vi "WaitBallOrientSkill.vi"(6 "Role ofRobotThat\nmake the pass":T1=enum."PassKicker", 8 "error in (no error)":errorcluster, 9 "Robot":refnum<class "Robot.lvclass">, 10 "Game":refnum<class "Game.lvclass">, 11 "WaitBallOrientSkill in":refnum<class "WaitBallOrientSkill.lvclass">) -> (0 "error out":errorcluster, 2 "robot out":refnum<class "Robot.lvclass">, 3 "WaitBallOrientSkill out":refnum<class "WaitBallOrientSkill.lvclass">)   [LabVIEW 2024, in "WaitBallOrientSkill.lvclass"]
uses:
  WaitBallOrientSkill.lvclass
  Robot_class/Robot.lvclass
  C:/Users/moise/Documents/GitHub/SSL_AI/Object_class/Object.lvclass
  Game_class/Game.lvclass
  Robot_class/roles.ctl
  Object_class/Object.lvclass/Object.ctl
  Game_class/Game.lvclass/Game.ctl
  Team_class/Team.lvclass/Team.ctl
  Robot_class/Robot.lvclass/Robot.ctl
  Game_class/Read BallRef.vi
  Game_class/Read Utilities.lvclass.vi
  Game_class/Read FieldRef.vi
  Game_class/Read OffensiveTeam.vi
  Team_class/Read RobotRef.vi
  Object_class/Read x.vi
  Object_class/Read y.vi
  Robot_class/Read orientation.vi
  Robot_class/Write dest_x.vi
  Robot_class/Write dest_y.vi
  Robot_class/Write dest_orientation.vi
  Ally_class/Ally.lvclass
  C:/Users/moise/Documents/GitHub/SSL_AI/Team_class/Team.lvclass
  Ball_class/Ball.lvclass
  Utilities_class/Utilities.lvclass
  Field_class/Field.lvclass
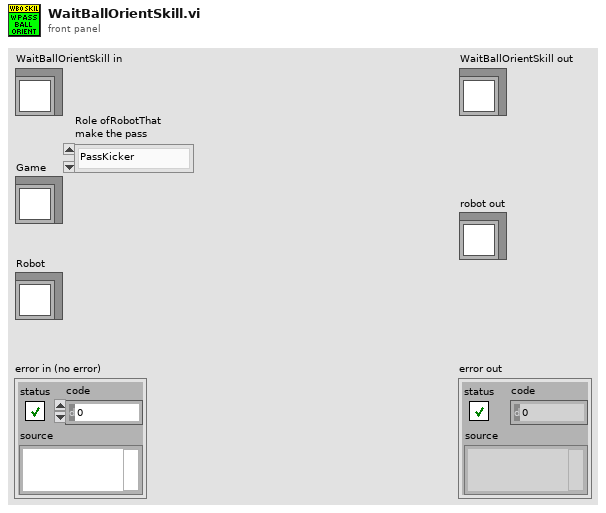
[diagram p1: front panel]
types:
  T1 = typedef "roles.ctl" = enum16{"SimpleBallPlacement", "BallPlacementAllyPasser", "BallPlacementAllyReceiver", "BallPlacementEnemy", "5Robots5th", "PassBestReceiver", "5Robots4th", "5Robots3rd", "5Robots2nd", "5Robots1st", "PassBestRobot", "WaitPass", "ABCThirdKicker", "ABCFirstKicker", "ABCSecondKicker", "Tabler", "TableFinalizer", "PrepareRollToPassRoller", "PrepareRollToPassReceiver", "SimplePassRoll", "SimplePassRollReceiver", "PenaltyDefense", "PreparePassReceiver 2", "PreparePassReceiver 1", "PassObserver", "Timeout", "Goto", "ZigZag", "None", "BallOutOfField", "DefenderArea", "Duelist", "AttackerStop", "FollowAttacker", "KeeperRole", "KickPenalty", "AttackerAimGoal", "AttackerBlock", "Marker", "Halt", "Shoot", "PassKicker", "PassReceiver", "TestRole", "PenaltyAttacker"}
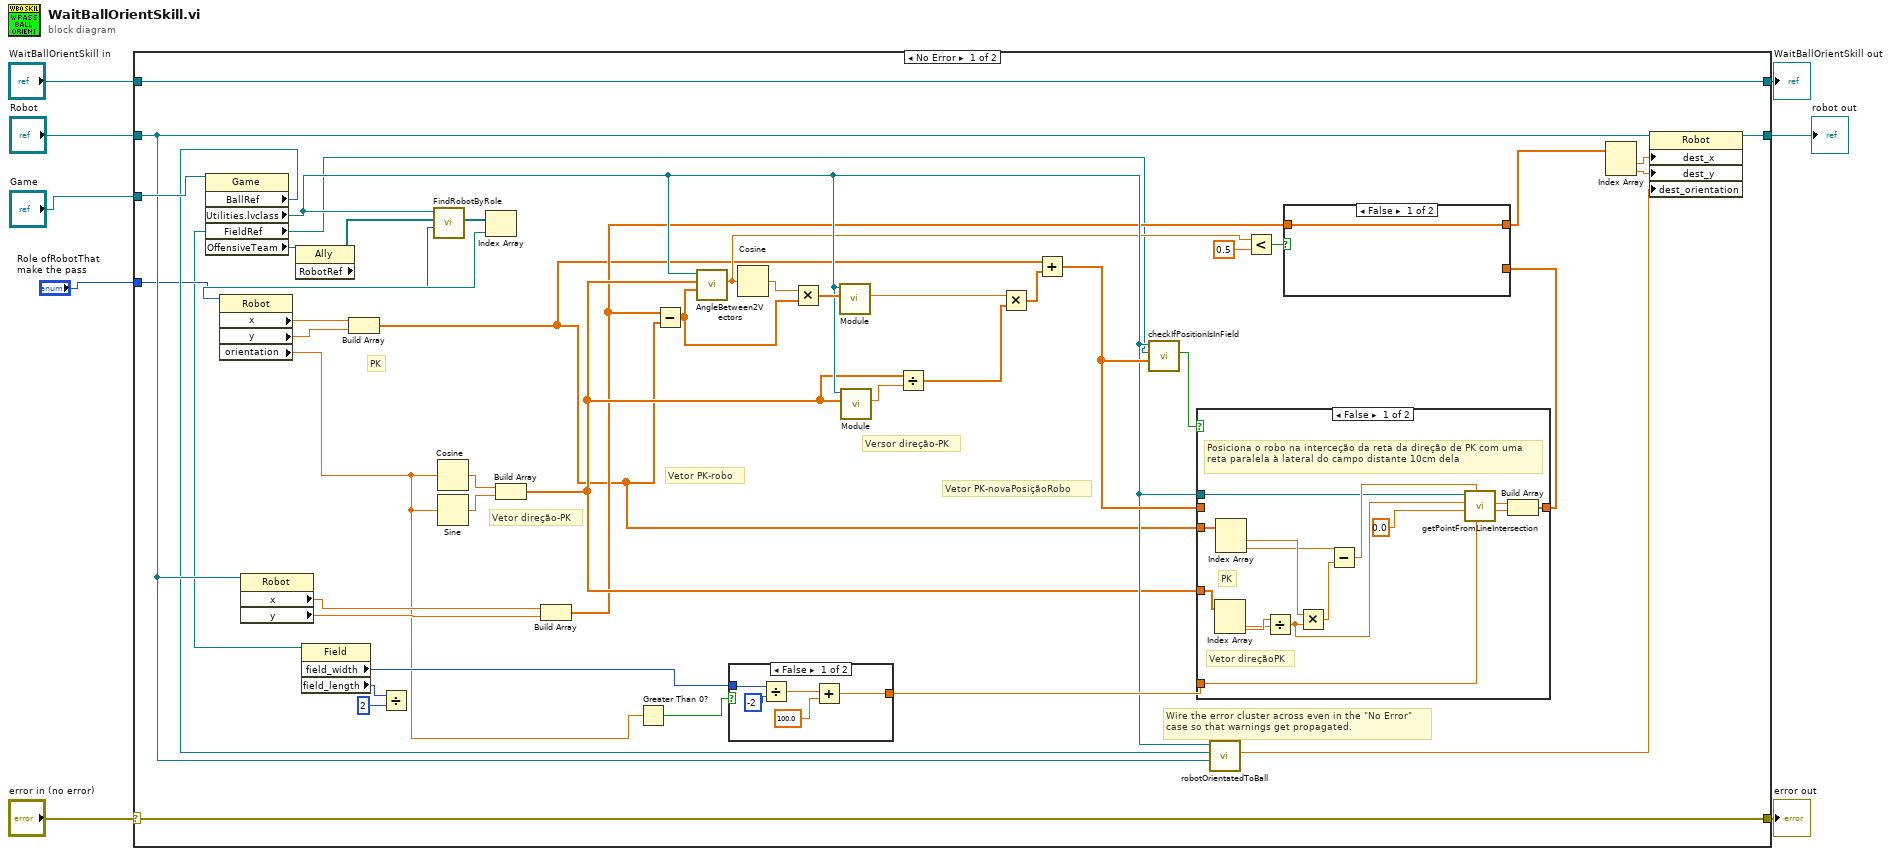
[diagram p0: block diagram]
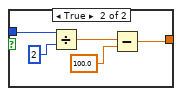
[diagram p4: hidden frame]
diagram:
  n1 = case shown="No Error" "error in (no error)" {
    selector: "error in (no error)" -> [w52 w83]
    tunnel: [w52 w83] -> w7
    tunnel: [w53 w82] -> w5
    tunnel: "WaitBallOrientSkill in" -> [w53 w82]
    tunnel: "Robot" -> [w29 _]
    tunnel: [w34 _] -> w3
    tunnel: "Game" -> [w30 _]
    tunnel: "Role ofRobotThat\nmake the pass" -> [w15 _]
    frame No Error {
      # "Versor direção-PK"
      # "PK"
      # "Vetor direção-PK"
      # "Vetor PK-novaPosiçãoRobo"
      # "Vetor PK-robo"
      # "Wire the error cluster across even in the \"No Error\"\ncase so that warnings get propagated."
      n2 = property class="Game"(reference=w30) -> ("BallRef"=w16:refnum<class "Ball.lvclass">, "Utilities.lvclass"=w25:refnum<class "Utilities.lvclass">, "FieldRef"=w13:refnum<class "Field.lvclass">, "OffensiveTeam"=w40:refnum<class "Ally.lvclass">)  [unwired: 1 in, 2 out]
      n3 = property class="Robot"(reference=w29) -> ("x"=w51:dbl, "y"=w50:dbl)  [unwired: 1 in, 2 out]
      n4 = property class="Ally"(reference=w40) -> ("RobotRef"=w39:refnum<class "Robot.lvclass">[])  [unwired: 1 in, 2 out]
      n5 = property class="Field"(reference=w13) -> ("field_width"=w44:i32, "field_length"=w12:i32)  [unwired: 1 in, 2 out]
      n6 = Divide(x=w12, y=2) -> ()  [unwired: 1 out]
      n7 = call "FindRobotByRole.vi"("role"=w15, "RobotRef"=w39, "Utilities in"=w25) -> ("Robots"=w37:refnum<class "Robot.lvclass">[])  [unwired: 5 in, 3 out]
      n8 = Index Array(array=w37) -> (element=w38:refnum<class "Robot.lvclass">)  [unwired: 1 in]
      n9 = property class="Robot"(reference=w38) -> ("x"=w36:dbl, "y"=w35:dbl, "orientation"=w31:dbl)  [unwired: 1 in, 2 out]
      n10 = Build Array(w36, w35) -> (w10:dbl[])
      n11 = Cosine(x=w31) -> (cos(x)=w33:dbl)
      n12 = Sine(x=w31) -> (sin(x)=w32:dbl)
      n13 = Build Array(w33, w32) -> (w23:dbl[])
      n14 = Build Array(w51, w50) -> (w19:dbl[])
      n15 = Greater Than 0?(x=w31) -> (x > 0?=w45:bool)
      n16 = Subtract(x=w19, y=w10) -> (x-y=w49:dbl[])
      n17 = call "AngleBetween2Vectors.vi"("Array 1"=w49, "Array 2"=w23, "Utilities in"=w25) -> ("angleInRadians(default)"=w20:dbl)  [unwired: 5 in, 3 out]
      n18 = case shown="False" w45 {
        tunnel: w44 -> [w75 w81]
        tunnel: [w74 w79] -> w43
        frame False {
          n19 = Divide(x=w75, y=-2) -> (x/y=w73:dbl)
          n20 = Add(x=w73, y=100.0) -> (x+y=w74:dbl)
        }
        frame True {
          n21 = Divide(x=w81, y=2) -> (x/y=w78:dbl)
          n22 = Subtract(x=w78, y=100.0) -> (x-y=w79:dbl)
        }
      }
      n23 = Cosine(x=w20) -> (cos(x)=w48:dbl)
      n24 = Multiply(x=w48, y=w49) -> (x*y=w28:dbl[])
      n25 = call "Module.vi"("2D vector"=w28, "Utilities in"=w25) -> ("Modulo"=w26:dbl)  [unwired: 7 in, 2 out]
      n26 = call "Module.vi"("2D vector"=w23, "Utilities in"=w25) -> ("Modulo"=w22:dbl)  [unwired: 7 in, 2 out]
      n27 = Divide(x=w23, y=w22) -> (x/y=w24:dbl[])
      n28 = Multiply(x=w26, y=w24) -> (x*y=w27:dbl[])
      n29 = Add(x=w10, y=w27) -> (x+y=w46:dbl[])
      n30 = call "checkIfPositionIsInField.vi"("Position"=w46, "FieldRef"=w13, "Utilities in"=w25) -> ("Position Is In Field?"=w47:bool)  [unwired: 4 in, 4 out]
      n31 = case shown="False" w47 {
        tunnel: w46 -> [_ w71]
        tunnel: [w68 w71] -> w17
        tunnel: w43 -> [w66 _]
        tunnel: w10 -> [w65 _]
        tunnel: w23 -> [w64 _]
        tunnel: w25 -> [w56 _]
        frame False {
          # "PK"
          # "Vetor direçãoPK"
          # "Posiciona o robo na interceção da reta da direção de PK com uma reta paralela à lateral do campo distante 10cm dela"
          n32 = Index Array(array=w64) -> (element #1=w62:dbl, element #2=w63:dbl)  [unwired: 2 in]
          n33 = Index Array(array=w65) -> (element #1=w61:dbl, element #2=w60:dbl)  [unwired: 2 in]
          n34 = Divide(x=w63, y=w62) -> (x/y=w57:dbl)
          n35 = Multiply(x=w61, y=w57) -> (x*y=w59:dbl)
          n36 = Subtract(x=w60, y=w59) -> (x-y=w58:dbl)
          n37 = call "getPointFromLineIntersection.vi"("b2"=w66, "b1"=w58, "a2"=0.0, "a1"=w57, "Utilities in"=w56) -> ("y_intersection"=w69:dbl, "x_intersection"=w70:dbl)  [unwired: 3 in, 2 out]
          n38 = Build Array(w70, w69) -> (w68:dbl[])
        }
        frame True {
        }
      }
      n39 = call "robotOrientatedToBall.vi"("Robot"=w29, "BallRef"=w16, "Utilities in"=w25) -> ("Orientation"=w9:dbl)  [unwired: 6 in, 2 out]
      n40 = Less?(x=w20, y=0.5) -> (x < y?=w14:bool)
      n41 = case shown="False" w14 {
        tunnel: w19 -> [w54 _]
        tunnel: [w54 w55] -> w18
        tunnel: w17 -> [_ w55]
        frame False {
        }
        frame True {
        }
      }
      n42 = Index Array(array=w18) -> (element #1=w42:dbl, element #2=w41:dbl)  [unwired: 2 in]
      n43 = property class="Robot"(reference=w29, "dest_x"=w42, "dest_y"=w41, "dest_orientation"=w9) -> (reference out=w34:refnum<class "Robot.lvclass">)  [unwired: 1 in, 1 out]
    }
    frame Error {
    }
  }
  "error out" <- w7
  "WaitBallOrientSkill out" <- w5
  "robot out" <- w3
